vi "Anotate Image.vi"(10 "Sorted Array":T2(array[cluster]), 11 "Image Refnum in":T1) -> (3 "Image Refnum out":T1)   [LabVIEW 2012]
uses:
  <vilib>/vision/Image Controls.llb/IMAQ Image.ctl
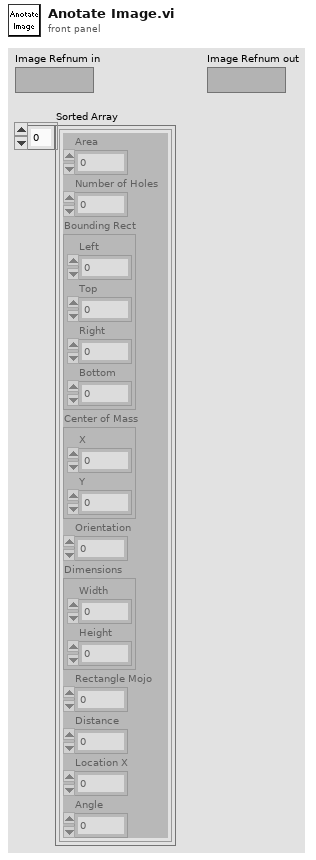
[diagram p1: front panel]
types:
  T1 = typedef "IMAQ Image.ctl" = refnum<image>
  T2 = cluster{"Area":dbl, "Number of Holes":dbl, "Bounding Rect":cluster{"Left":dbl, "Top":dbl, "Right":dbl, "Bottom":dbl}, "Center of Mass":cluster{"X":dbl, "Y":dbl}, "Orientation":dbl, "Dimensions":cluster{"Width":dbl, "Height":dbl}, "Rectangle Mojo":dbl, "Distance":dbl, "Location X":dbl, "Angle":dbl}[]
  T3 = cluster{"Left":i32, "Top":i32, "Right":i32, "Bottom":i32}
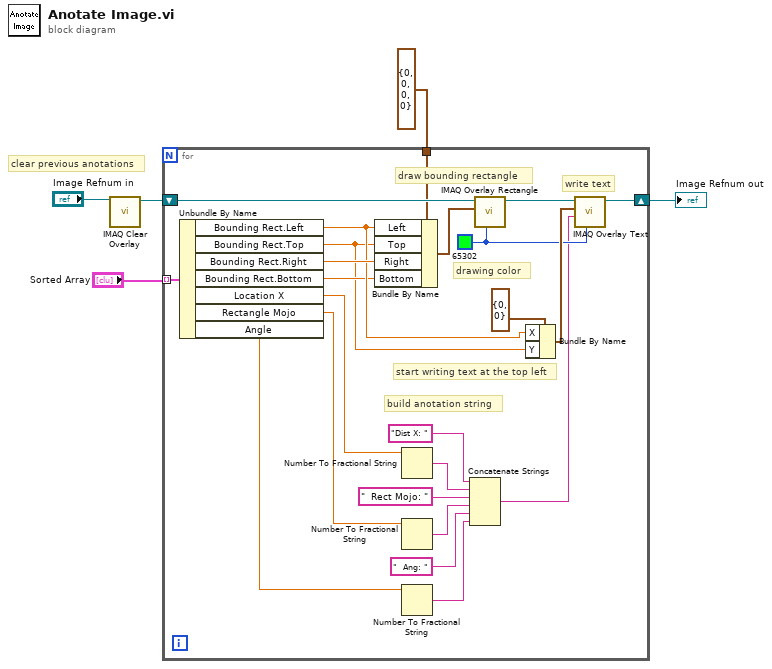
[diagram p0: block diagram]
diagram:
  # "clear previous anotations"
  n1 = call "IMAQ Clear Overlay"("Image"="Image Refnum in") -> ("Image Out"=w4:T1)  [unwired: 9 in, 1 out]
  n2 = for {
    tunnel: "Sorted Array" -> [w19] mode=indexing
    shift-right: [w13] -> w2
    shift-left: w4 -> [w12]
    tunnel: T3 {"Left"=0, "Top"=0, "Right"=0, "Bottom"=0} ("Rectangle") -> [w8]
    w20 = u32 65302 ("Color")
    # "draw bounding rectangle"
    # "build anotation string"
    # "start writing text at the top left"
    # "write text"
    # "drawing color"
    n3 = Unbundle By Name(w19) -> ("Bounding Rect.Left"=w23:dbl, "Bounding Rect.Top"=w21:dbl, "Bounding Rect.Right"=w27:dbl, "Bounding Rect.Bottom"=w22:dbl, "Location X"=w6:dbl, "Rectangle Mojo"=w18:dbl, "Angle"=w9:dbl)
    n4 = Bundle By Name(cluster=w8, "Left"=w23, "Top"=w21, "Right"=w27, "Bottom"=w22) -> (w28:T3)
    n5 = Number To Fractional String(number=w6) -> (F-format string=w17:string)  [unwired: 3 in]
    n6 = Number To Fractional String(number=w18) -> (F-format string=w15:string)  [unwired: 3 in]
    n7 = Number To Fractional String(number=w9) -> (F-format string=w10:string)  [unwired: 3 in]
    n8 = Concatenate Strings("Dist X: ", w17, "  Rect Mojo: ", w15, "  Ang: ", w10) -> (w14:string)
    n9 = call "IMAQ Overlay Rectangle"("Color"=w20, "Rectangle"=w28, "Image"=w12) -> ("Image Out"=w26:T1)  [unwired: 3 in, 5 out]
    n10 = Bundle By Name(cluster=cluster{"X":i32, "Y":i32} {"X"=0, "Y"=0} ("Origin"), "X"=w23, "Y"=w21) -> (w24:cluster{"X":i32, "Y":i32})
    n11 = call "IMAQ Overlay Text"("Text Color (black)"=w20, "String"=w14, "Origin"=w24, "Image"=w26) -> ("Image Out"=w13:T1)  [unwired: 6 in, 1 out]
  }
  "Image Refnum out" <- w2
